vi "Generate Exit Event.vi"(8 "error in (no error)":errorcluster) -> (0 "error out":errorcluster)   [LabVIEW 2020, in "WebServiceImporter.lvlib" / "Main Panel.lvlib" / "Events.lvlib"]
uses:
  <vilib>/Platform/WebService/Main Panel/Events/Events.lvlib
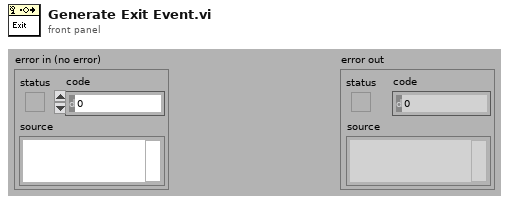
[diagram p1: front panel]
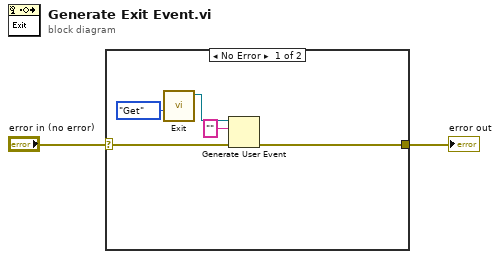
[diagram p0: block diagram]
diagram:
  n1 = case shown="No Error" "error in (no error)" {
    selector: "error in (no error)" -> [w7 w8]
    tunnel: [w3 w8] -> w1
    frame No Error {
      n2 = call <vilib>:"Exit.vi"("Operation"=enum16{"Get", "Set"}."Get") -> ("user event (out)"=w5:refnum<user-event>)  [unwired: 10 in]
      n3 = Generate User Event(user event=w5, event data cluster="" ("event data"), error in=w7) -> (error out=w3:errorcluster)  [unwired: 1 in, 1 out]
    }
    frame Error {
    }
  }
  "error out" <- w1
